vi "InfiniiumGetHisto.vi"(1 "Numeric":i32=10000, 2 "VISA resource name":refnum<visa-resource-name>) -> (0 "Array":dbl[](array[numeric]))   [LabVIEW 2014]
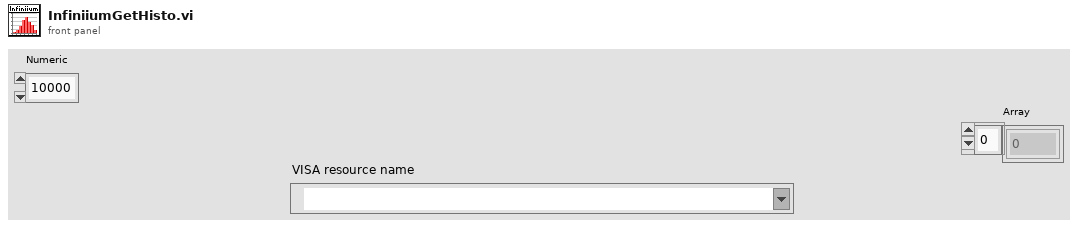
[diagram p1: front panel]
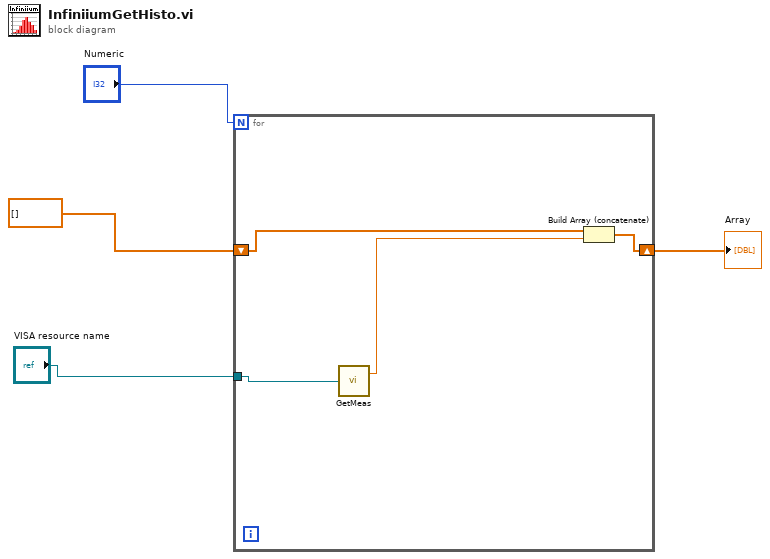
[diagram p0: block diagram]
diagram:
  n1 = for {
    N: "Numeric" -> [_]
    tunnel: "VISA resource name" -> [w6]
    shift-right: [w7] -> w1
    shift-left: dbl[] [] -> [w8]
    n2 = call "GetMeas.vi"("VISA resource name"=w6) -> ("Measure"=w5:dbl)  [unwired: 1 out]
    n3 = Build Array (concatenate)(w8, w5) -> (w7:dbl[])
  }
  "Array" <- w1
